vi "TemperatureVI.vi"(9 "Enable \nTemperature":bool, 10 "Voltage":dbl, 11 "Relative Humidity":dbl) -> (2 "Temperature":dbl, 3 "Humidity with\nTemperature Adjustment":dbl)   [LabVIEW 2018]
uses:
  <vilib>/express/express shared/transition.llb/Dynamic To Waveform Array.vi
  <vilib>/express/express arith-compare/Formula/Block/exnFormulaBlock how many pts in the wave.vi
  <vilib>/express/express shared/ex_Modify Signal Name.vi
  <vilib>/express/express shared/transition.llb/Waveform Array To Dynamic.vi
  <vilib>/express/express arith-compare/Formula/XNode/ExpressFormulaBlockNode.xnode
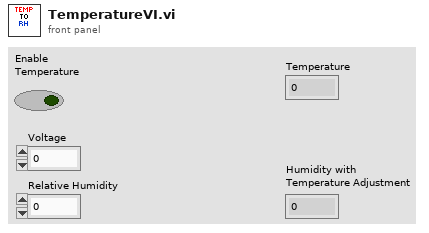
[diagram p1: front panel]
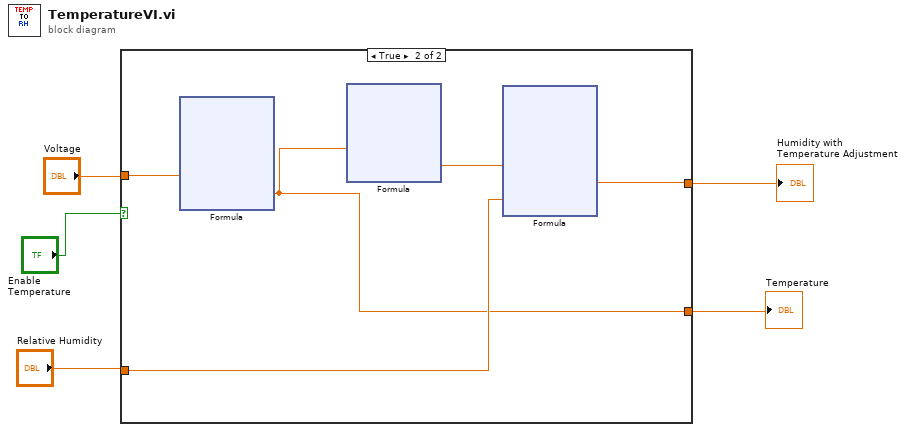
[diagram p0: block diagram]
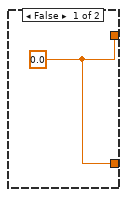
[diagram p2: hidden frame]
diagram:
  n1 = case shown="True" "Enable \nTemperature" {
    tunnel: "Voltage" -> [_ w11]
    tunnel: "Relative Humidity" -> [_ w9]
    tunnel: [w6 w7] -> w1
    tunnel: [w6 w8] -> w2
    frame False {
      w6 = 0.0
    }
    frame True {
      n2 = xnode "Formula"("V"=w11) -> ("Result"=w8:dbl)  [unwired: 1 in, 1 out]
      n3 = xnode "Formula"("F"=w8) -> ("Result"=w10:dbl)  [unwired: 1 in, 1 out]
      n4 = xnode "Formula"("C"=w10, "RH"=w9) -> ("Result"=w7:dbl)  [unwired: 1 in, 1 out]
    }
  }
  "Humidity with\nTemperature Adjustment" <- w1
  "Temperature" <- w2
